vi "ConfigDataSendTimeout.vi"(7 "clear":bool, 8 "error in (no error)":errorcluster, 10 "timeout (45)":dbl=45.0, 11 "Qbus in":refnum<class "Qbus.lvclass">) -> (0 "error out":errorcluster, 3 "Qbus out":refnum<class "Qbus.lvclass">)   [LabVIEW 2017, in "ServerComm.lvlib"]
uses:
  <vilib>/addons/InsightCM/Devices/Shared/Common/ServerComm/ServerComm.lvlib
  <vilib>/addons/Qbus/Qbus.lvclass
  <vilib>/addons/TimerProcess/controls/taskType.ctl
  <vilib>/addons/TimerProcess/TimerProcess.lvlib
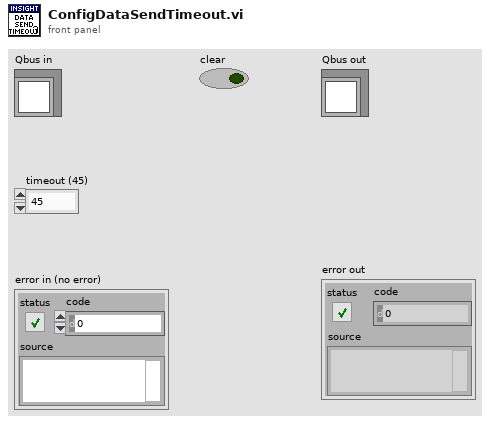
[diagram p1: front panel]
types:
  T1 = typedef "TimerProcess.lvlib/taskType.ctl" = enum16{"single", "repeat"}
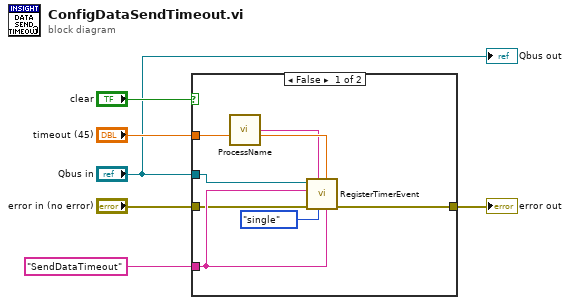
[diagram p0: block diagram]
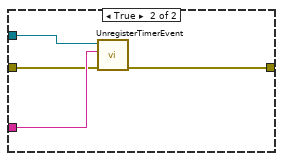
[diagram p2: hidden frame]
diagram:
  n1 = case shown="False" "clear" {
    tunnel: "timeout (45)" -> [w13 _]
    tunnel: "Qbus in" -> [w12 w17]
    tunnel: "SendDataTimeout" ("CallBackAction") -> [w11 w16]
    tunnel: "error in (no error)" -> [w8 w15]
    tunnel: [w7 w14] -> w2
    frame False {
      n2 = call <vilib>:"ProcessName.vi"() -> ("process name"=w10:string)  [unwired: 5 in]
      n3 = call <vilib>:"RegisterTimerEvent.vi"("timer task name"=w11, "interval (sec)"=w13, "type"=taskType."single", "process name"=w10, "error in (no error)"=w8, "callback action"=w11, "qbus in"=w12) -> ("error out"=w7:errorcluster)  [unwired: 3 in, 1 out]
    }
    frame True {
      n4 = call <vilib>:"UnregisterTimerEvent.vi"("error in (no error)"=w15, "timer task name"=w16, "qbus in"=w17) -> ("error out"=w14:errorcluster)  [unwired: 7 in, 1 out]
    }
  }
  "error out" <- w2
  "Qbus out" <- "Qbus in"
